vi "Inalfa SCU LIN Message to Move.vi"(10 "Communication Type":T1, 11 "Motion":T2) -> (3 "Have Swtich?":bool)   [LabVIEW 2018]
uses:
  02.Type Def's/All Motions.ctl
  02.Type Def's/All Communication Types.ctl
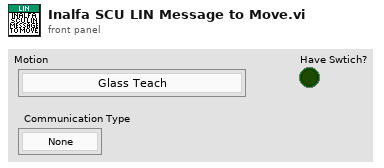
[diagram p1: front panel]
types:
  T1 = typedef "All Communication Types.ctl" = enum16{"None", "CAN", "RS 232", "RS 232 LIN", "GM LIN", "SnT LIN", "K Line", "Robel CAN", "P42M-Continental", "Inalfa SCU LIN", "Spare 3"}
  T2 = typedef "All Motions.ctl" = enum16{"Glass Teach", "Glass Slide Open", "Glass Slide Close", "Glass Vent Open", "Glass Vent Close", "Sunshade Teach", "Sunshade Open", "Sunshade Close", "Idle", "Sunshade Open 2", "Sunshade Close 2", "Glass Slide Open Sunshade Open", "Glass Slide Open Sunshade Close", "Glass Slide Close Sunshade Open", "Glass Slide Close Sunshade Close", "Glass Vent Open Sunshade Open", "Glass Vent Open Sunshade Close", "Glass Vent Close Sunshade Open", "Glass Vent Close Sunshade Close", "Express Glass Slide Open", "Express Glass Slide Close", "Express Glass Vent Open", "Express Glass Vent Close", "Express Sunshade Open", "Express Sunshade Close", "Express Sunshade Open 2", "Express Sunshade Close 2", "Express Glass Slide Open Sunshade Open", "Express Glass Slide Open Sunshade Close", "Express Glass Slide Close Sunshade Open", "Express Glass Slide Close Sunshade Close", "Express Glass Vent Open Sunshade Open", "Express Glass Vent Open Sunshade Close", "Express Glass Vent Close Sunshade Open", "Express Glass Vent Close Sunshade Close", "Goto Position Glass", "Goto Position Sunshade", "Sunshade Teach 2"}
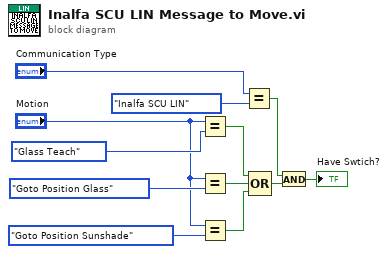
[diagram p0: block diagram]
diagram:
  n1 = Equal?(x="Motion", y=All_Motions."Glass Teach") -> (x = y?=w6:bool)
  n2 = Equal?(x="Motion", y=All_Motions."Goto Position Glass") -> (x = y?=w5:bool)
  n3 = Equal?(x="Motion", y=All_Motions."Goto Position Sunshade") -> (x = y?=w4:bool)
  n4 = Equal?(x="Communication Type", y=All_Communication_Types."Inalfa SCU LIN" ("Communication Type")) -> (x = y?=w12:bool)
  n5 = Compound Arithmetic op=OR(w6, w5, w4) -> (w3:bool)
  n6 = And(x=w12, y=w3) -> (x .and. y?=→"Have Swtich?":bool)
